vi "GetParam.vi"(8 "error in (no error)":errorcluster caption="entrée d'erreur (pas d'erreur)", 11 "Polynomial_kernel.lvclass":refnum<class "Polynomial_kernel.lvclass">) -> (0 "error out":errorcluster caption="sortie d'erreur", 2 "polynomial_kernel":T1={"degree"=3, "gamma"="None", "coef0"=1.0}, 3 "Polynomial_kernel.lvclass":refnum<class "Polynomial_kernel.lvclass">)   [LabVIEW 2020, in "Polynomial_kernel.lvclass"]
doc: "Get Parameters"
uses:
  Polynomial_kernel.lvclass
  Polynomial_kernel.lvclass/Polynomial_kernel.ctl
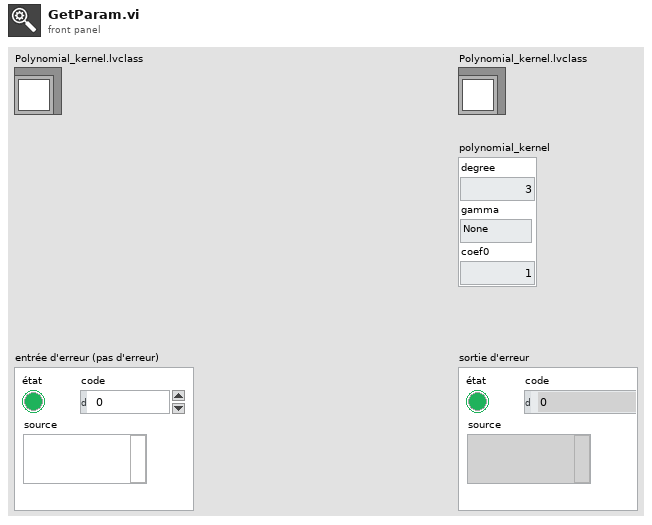
[diagram p1: front panel]
types:
  T1 = cluster{"degree":i32, "gamma":string, "coef0":dbl}
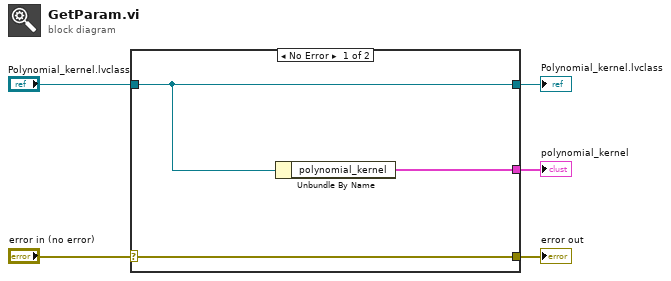
[diagram p0: block diagram]
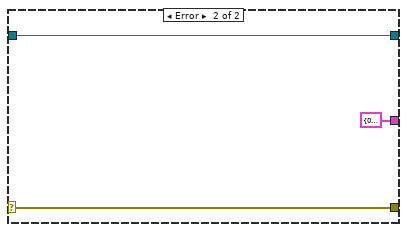
[diagram p2: hidden frame]
diagram:
  n1 = case shown="No Error" "error in (no error)" {
    selector: "error in (no error)" -> [w8 w10]
    tunnel: [w8 w10] -> w4
    tunnel: [w7 w11] -> w2
    tunnel: "Polynomial_kernel.lvclass" -> [w7 w11]
    tunnel: [w6 T1 {"degree"=0, "gamma"="", "coef0"=0.0} ("polynomial_kernel")] -> w1
    frame No Error {
      n2 = Unbundle By Name(w7) -> ("polynomial_kernel"=w6:T1)
    }
    frame Error {
    }
  }
  "error out" <- w4
  "Polynomial_kernel.lvclass" <- w2
  "polynomial_kernel" <- w1
